vi "dvotZFTConstants.vi"() -> ()   [LabVIEW 2012]
panel:
  out "YAMADA_ET_AL_2007":dbl=2.0
  out "RAHN_ET_AL_2004":dbl=1.0
  out "KETCHAM_2012":dbl
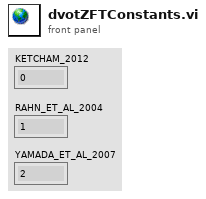
[diagram p1: front panel]
diagram:
